vi "Begin.vi"(8 "error in (no error)":errorcluster, 11 "GrabberWheels in":refnum<class "GrabberWheels.lvclass">) -> (0 "error out":errorcluster, 3 "GrabberWheels out":refnum<class "GrabberWheels.lvclass">)   [LabVIEW 2013, in "GrabberWheels.lvclass"]
uses:
  GrabberWheels.lvclass
  <vilib>/Rock Robotics/WPI/CAN/Jaguar/SubVIs/WPI_CANJaguar_ControlMode.ctl
  System/System.lvclass
  <vilib>/Rock Robotics/WPI/MotorControl/WPI_MotorControlOpenCANJaguar.vi
panel:
  in  "Device Number":u8=7
  in  "Control Mode":T1
  in  "Invert":bool=TRUE
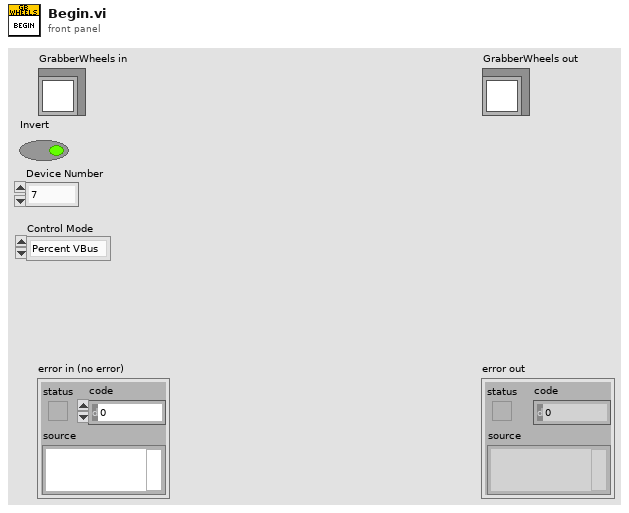
[diagram p1: front panel]
types:
  T1 = typedef "WPI_CANJaguar_ControlMode.ctl" = enum8{"Percent VBus", "Current", "Speed", "Position", "Voltage"}
  T2 = typedef "WPI_MotorControlDeviceRef.ctl" = cluster{"DeviceStatus":errorcluster, "Type":enum16{"PWM", "CAN"}, "PWM":cluster{"Digital Module":T3, "PWM Channel":T4, "DeadBand":T5}, "CAN":cluster{"Device Number":u8, "Control Mode":T1, "Semaphore":T6, "Max Vout":dbl}, "Invert":bool, "TransformRef":T7, "InvTransformRef":T7}
  T3 = typedef "FPGA_TypedefDigitalModule.ctl" = enum16{"Digital Module 1", "Digital Module 2"}
  T4 = typedef "FPGA_DIOPWMChannel.ctl" = enum8{"PWM 1", "PWM 2", "PWM 3", "PWM 4", "PWM 5", "PWM 6", "PWM 7", "PWM 8", "PWM 9", "PWM 10", "Invalid"}
  T5 = typedef "WPI_PWMDeadband.ctl" = cluster{"Name":string, "maxPositivePwm":i32, "minPositivePwm":i32, "centerPwm":i32, "maxNegativePwm":i32, "minNegativePwm":i32, "angularRange":u16}
  T6 = typedef "Semaphore RefNum" = refnum<k1>
  T7 = typedef "WPI_PWMTransform_ConPane.ctl" = refnum<vi>
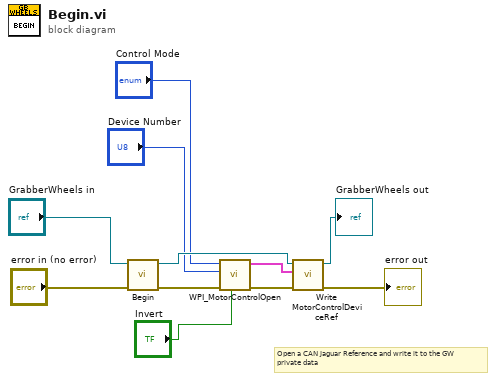
[diagram p0: block diagram]
diagram:
  # "Open a CAN Jaguar Reference and write it to the GW \nprivate data"
  n1 = call-parent "Begin.vi"("error in (no error)"="error in (no error)", "System in"="GrabberWheels in") -> ("error out"=w2:errorcluster, "System out"=w9:refnum<class "GrabberWheels.lvclass">)  [unwired: 8 in]
  n2 = call-poly <vilib>:"WPI_MotorControlOpen.vi"("Invert"="Invert", "error in (no error)"=w2, "Device Number"="Device Number", "Control Mode"="Control Mode") -> ("error out"=w1:errorcluster, "MotorControlDeviceRef"=w6:T2)  [unwired: 6 in]
  n3 = call-dynamic "Write MotorControlDeviceRef.vi"("error in (no error)"=w1, "MotorControlDeviceRef"=w6, "GrabberWheels in"=w9) -> ("error out"=→"error out":errorcluster, "GrabberWheels out"=→"GrabberWheels out":refnum<class "GrabberWheels.lvclass">)  [unwired: 7 in]
